vi "BuildConfigWord.vi"(11 "NewVal":T1) -> (3 "string":string)   [LabVIEW 2020]
uses:
  Adafruit NAU7802 24bit Strain Gauge.lvclass/Adafruit NAU7802 24bit Strain Gauge.ctl
  ConfigData.ctl
  NAU7802PGA.ctl
  Adafruit NAU7802 24bit Strain Gauge.lvclass
  NAU7802LDOVoltage.ctl
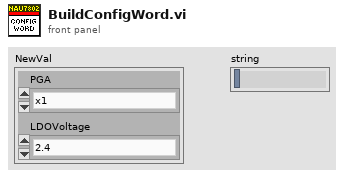
[diagram p1: front panel]
types:
  T1 = typedef "ConfigData.ctl" = cluster{"PGA":T2, "LDOVoltage":T3}
  T2 = typedef "CTI-Peripheral.lvlib/Adafruit NAU7802 24bit Strain Gauge.lvclass/NAU7802PGA.ctl" = enum16{"x1", "x2", "x4", "x8", "x16", "x32", "x64", "x128"}
  T3 = typedef "CTI-Peripheral.lvlib/Adafruit NAU7802 24bit Strain Gauge.lvclass/NAU7802LDOVoltage.ctl" = enum16{"2.4", "2.7", "3.0", "3.3", "3.6", "3.9", "4.2", "4.5"}
  T4 = typedef "ADS1115Mux.ctl" = enum16{"Single AI0 - GND", "Single AI1 - GND", "Single AI2 - GND", "Single AI3 - GND"}
  T5 = typedef "ADS1115Mode.ctl" = enum16{"Continuous", "Single-Shot"}
  T6 = typedef "CTI-Peripheral.lvlib/Adafruit NAU7802 24bit Strain Gauge.lvclass/NAU7802DataRate.ctl" = enum16{"10 SPS", "20 SPS", "40 SPS", "80 SPS", "320 SPS"}
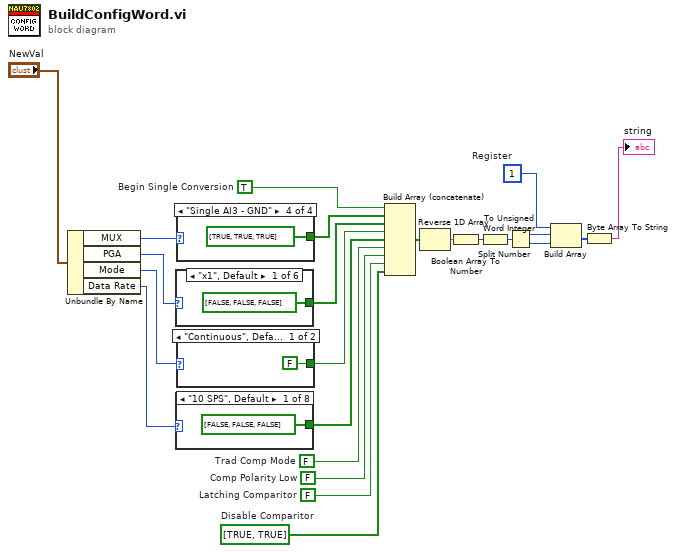
[diagram p0: block diagram]
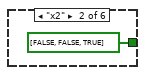
[diagram p2: hidden frame]
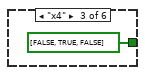
[diagram p3: hidden frame]
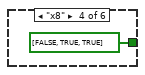
[diagram p4: hidden frame]
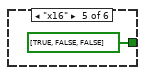
[diagram p5: hidden frame]
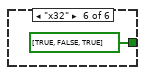
[diagram p6: hidden frame]
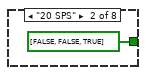
[diagram p7: hidden frame]
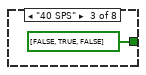
[diagram p8: hidden frame]
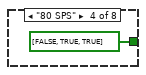
[diagram p9: hidden frame]
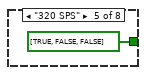
[diagram p10: hidden frame]
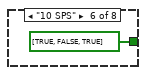
[diagram p11: hidden frame]
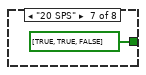
[diagram p12: hidden frame]
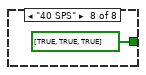
[diagram p13: hidden frame]
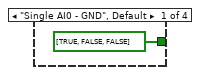
[diagram p14: hidden frame]
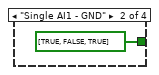
[diagram p15: hidden frame]
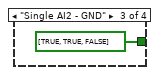
[diagram p16: hidden frame]
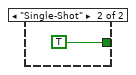
[diagram p17: hidden frame]
diagram:
  w1 = u8 1  # Register
  w15 = bool[] [TRUE, TRUE]  # Disable Comparitor
  w14 = FALSE  # Latching Comparitor
  w13 = FALSE  # Comp Polarity Low
  w12 = FALSE  # Trad Comp Mode
  w5 = TRUE  # Begin Single Conversion
  n1 = Unbundle By Name("NewVal") -> ("MUX"=w3:T4, "PGA"=w4:T2, "Mode"=w8:T5, "Data Rate"=w10:T6)
  n2 = case shown="\"x1\", Default" w4 {
    tunnel: [bool[] [FALSE, FALSE, FALSE] bool[] [FALSE, FALSE, TRUE] bool[] [FALSE, TRUE, FALSE] bool[] [FALSE, TRUE, TRUE] bool[] [TRUE, FALSE, FALSE] bool[] [TRUE, FALSE, TRUE]] -> w7
    frame "x1", Default {
    }
    frame "x2" {
    }
    frame "x4" {
    }
    frame "x8" {
    }
    frame "x16" {
    }
    frame "x32" {
    }
  }
  n3 = case shown="\"10 SPS\", Default" w10 {
    tunnel: [bool[] [FALSE, FALSE, FALSE] bool[] [FALSE, FALSE, TRUE] bool[] [FALSE, TRUE, FALSE] bool[] [FALSE, TRUE, TRUE] bool[] [TRUE, FALSE, FALSE] bool[] [TRUE, FALSE, TRUE] bool[] [TRUE, TRUE, FALSE] bool[] [TRUE, TRUE, TRUE]] -> w11
    frame "10 SPS", Default {
    }
    frame "20 SPS" {
    }
    frame "40 SPS" {
    }
    frame "80 SPS" {
    }
    frame "320 SPS" {
    }
    frame "10 SPS" {
    }
    frame "20 SPS" {
    }
    frame "40 SPS" {
    }
  }
  n4 = case shown="\"Single AI3 - GND\"" w3 {
    tunnel: [bool[] [TRUE, FALSE, FALSE] bool[] [TRUE, FALSE, TRUE] bool[] [TRUE, TRUE, FALSE] bool[] [TRUE, TRUE, TRUE]] -> w6
    frame "Single AI0 - GND", Default {
    }
    frame "Single AI1 - GND" {
    }
    frame "Single AI2 - GND" {
    }
    frame "Single AI3 - GND" {
    }
  }
  n5 = case shown="\"Continuous\", Default" w8 {
    tunnel: [FALSE TRUE] -> w9
    frame "Continuous", Default {
    }
    frame "Single-Shot" {
    }
  }
  n6 = Build Array (concatenate)(w5, w6, w7, w9, w11, w12, w13, w14, w15) -> (w16:bool[])
  n7 = Reverse 1D Array(array=w16) -> (reversed array=w21:bool[])
  n8 = Boolean Array To Number(Boolean array=w21) -> (number=w17:u32)
  n9 = To Unsigned Word Integer(number=w17) -> (unsigned 16bit integer=w18:u16)
  n10 = Split Number(x=w18) -> (hi(x)=w22:u8, lo(x)=w23:u8)
  n11 = Build Array(w1, w22, w23) -> (w19:u8[])
  n12 = Byte Array To String(unsigned byte array=w19) -> (string=→"string":string)
